vi "TcA01-008_NameObjectsWithUserCounter.vi"(1 "Input buffer":T3="1", 3 "Invocation info":T2, 5 "error in (no error)":errorcluster, 6 "Add log to result?":bool) -> (16 "Test Data":T1 {"Numeric Measurement" format="%.2f"}, 19 "error out":errorcluster)   [LabVIEW 2009]
doc: "Test case template."
uses:
  Shared/Support_InputBuffer.ctl
  Shared/Support_InvocationInfo.ctl
  Shared/Support_TestData.ctl
  <vilib>/addons/_AddQ/G#Object/utils/G#Object_CreateMethod.ctl
  TestClasses/G#BaseClass1_class/G#BaseClass1.lvclass
  TestClasses/G#SubClass1_class/G#SubClass1.lvclass
  <vilib>/addons/_AddQ/G#Object/G#Object.lvclass
panel:
  in  "Test name":string="TcA01-008 Name Objects With User Counter"
  out "Test result":bool
  out "Result":string
  # "Verify that objects can be named by a user counter."
  # "Sub test case"
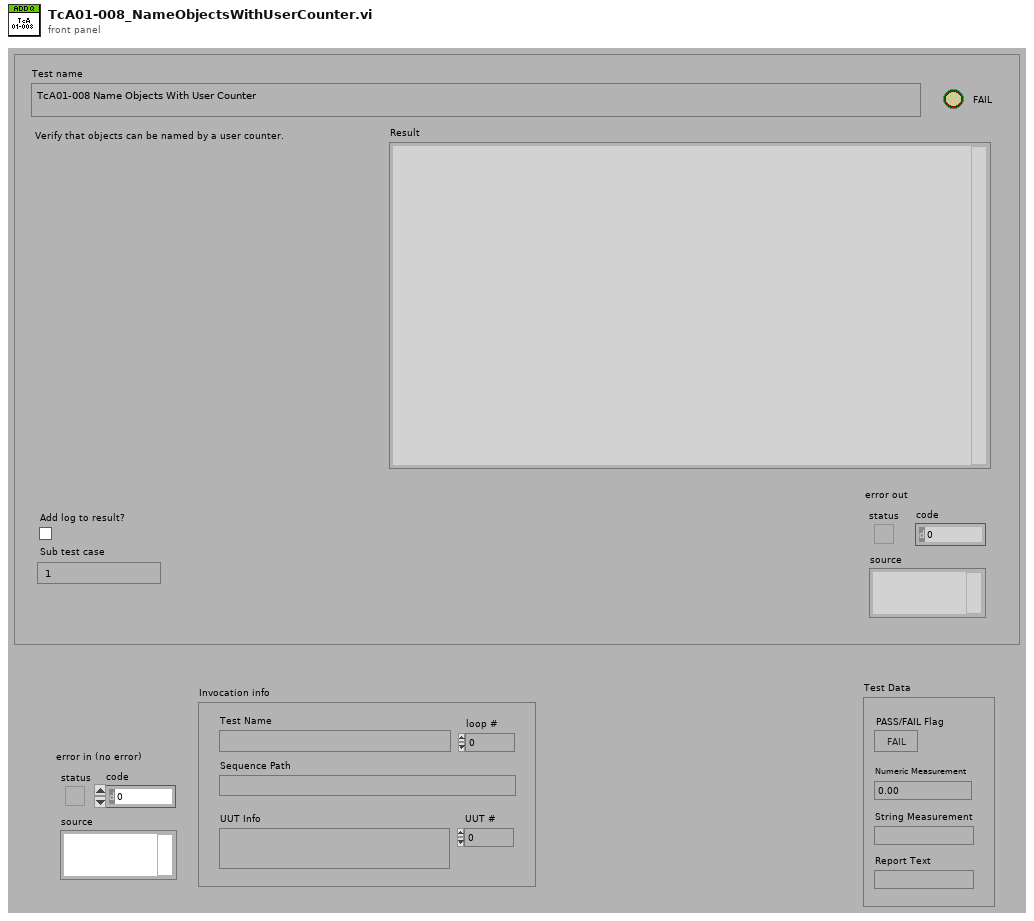
[diagram p1: front panel]
types:
  T1 = typedef "Support_TestData.ctl" = cluster{"PASS/FAIL Flag":bool, "Numeric Measurement":dbl, "String Measurement":string, "Report Text":string}
  T2 = typedef "Support_InvocationInfo.ctl" = cluster{"UUT #":i32, "loop #":i32, "UUT Info":string, "Test Name":string, "Sequence Path":path}
  T3 = typedef "Support_InputBuffer.ctl" = string
  T4 = typedef "G#Object.lvclass/G#Object_CreateMethod.ctl" = enum16{"Create", "Create or look up existing", "Look up existing"}
  T5 = typedef "Support_ResultType.ctl" = cluster{"Pass":bool, "Comment":string, "MeasurementValue":dbl}
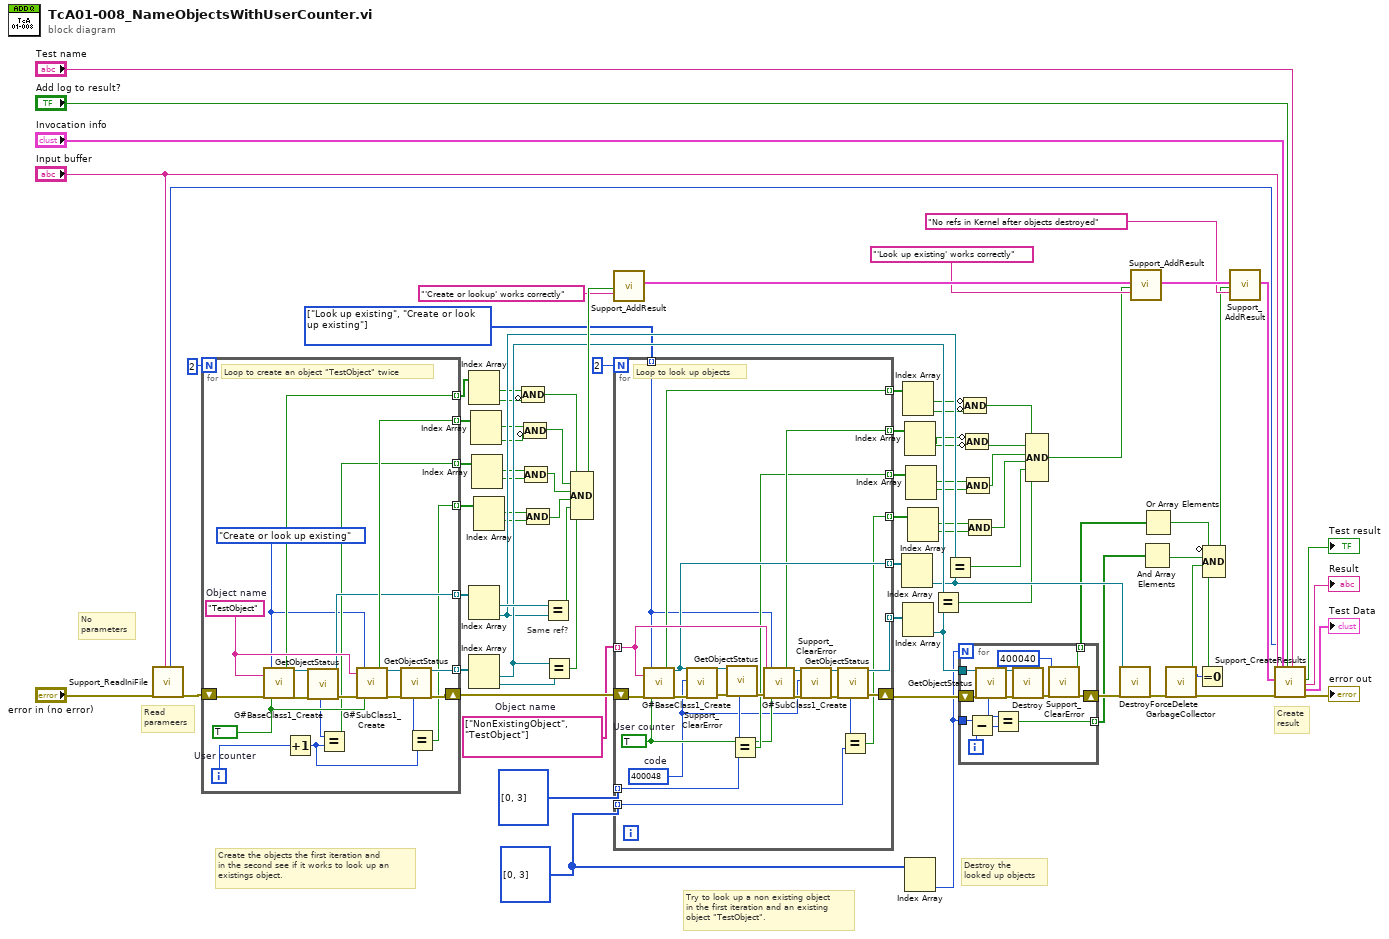
[diagram p0: block diagram]
diagram:
  w17 = T4[] [enum."Look up existing", enum."Create or look up existing"] items=["Create", "Create or look up existing", "Look up existing"]
  w11 = i32[] [0, 3]
  w31 = string[] ["NonExistingObject", "TestObject"]  # Object name
  # "Create the objects the first iteration and\nin the second see if it works to look up an\nexistings object."
  # "Try to look up a non existing object\nin the first iteration and an existing\nobject \"TestObject\"."
  # "Destroy the\nlooked up objects"
  # "Same ref?"
  # "No\nparameters"
  # "Create\nresult"
  # "Read\nparameers"
  n1 = call "Support_ReadIniFile.vi"("error in (no error)"="error in (no error)", "Sub test case"="Input buffer") -> ("Timer start"=w72:u32, "error out"=w71:errorcluster)  [unwired: 10 in, 6 out]
  n2 = for {
    N: 2 -> [_]
    shift-right: [w89] -> w57
    shift-left: w71 -> [w101]
    tunnel: [w94] -> w69 mode=indexing
    tunnel: [w90] -> w68 mode=indexing
    tunnel: [w98] -> w44 mode=indexing
    tunnel: [w97] -> w43 mode=indexing
    tunnel: [w86] -> w38 mode=indexing
    tunnel: [w83] -> w37 mode=indexing
    i -> [w87]
    w82 = G#Object_CreateMethod."Create or look up existing" ("create method")
    w99 = TRUE  # User counter
    w100 = "TestObject"  # Object name
    # "Loop to create an object \"TestObject\" twice"
    n3 = call "G#BaseClass1_Create.vi"("object name"=w100, "error in (no error)"=w101, "create method"=w82, "user counter"=w99) -> ("created new?"=w98:bool, "reference out"=w95:refnum<class "G#BaseClass1.lvclass">, "error out"=w96:errorcluster)  [unwired: 13 in]
    n4 = Increment(x=w87) -> (x+1=w84:i32)
    n5 = call-dynamic "GetObjectStatus.vi"("reference in"=w95, "error in (no error)"=w96) -> ("# of users?"=w88:i32, "reference out"=w94:refnum<class "G#BaseClass1.lvclass">, "error out"=w93:errorcluster)  [unwired: 6 in, 9 out]
    n6 = Equal?(x=w88, y=w84) -> (x = y?=w86:bool)
    n7 = call "G#SubClass1_Create.vi"("object name"=w100, "error in (no error)"=w93, "create method"=w82, "user counter"=w99) -> ("created new?"=w97:bool, "reference out"=w91:refnum<class "G#SubClass1.lvclass">, "error out"=w92:errorcluster)  [unwired: 13 in]
    n8 = call-dynamic "GetObjectStatus.vi"("reference in"=w91, "error in (no error)"=w92) -> ("# of users?"=w85:i32, "reference out"=w90:refnum<class "G#SubClass1.lvclass">, "error out"=w89:errorcluster)  [unwired: 6 in, 9 out]
    n9 = Equal?(x=w85, y=w84) -> (x = y?=w83:bool)
  }
  n10 = Index Array(array=w44) -> (element #1=w42:bool, element #2=w41:bool)  [unwired: 2 in]
  n11 = Index Array(array=w69) -> (element #1=w67:refnum<class "G#BaseClass1.lvclass">, element #2=w47:refnum<class "G#BaseClass1.lvclass">)  [unwired: 2 in]
  n12 = Index Array(array=w68) -> (element #1=w49:refnum<class "G#SubClass1.lvclass">, element #2=w66:refnum<class "G#SubClass1.lvclass">)  [unwired: 2 in]
  n13 = Index Array(array=w43) -> (element #1=w15:bool, element #2=w14:bool)  [unwired: 2 in]
  n14 = Index Array(array=w38) -> (element #1=w40:bool)  [unwired: 2 in, 1 out]
  n15 = Index Array(array=w37) -> (element #1=w39:bool)  [unwired: 2 in, 1 out]
  n16 = Compound Arithmetic op=AND(w42, invert w41) -> (w36:bool)
  n17 = Compound Arithmetic op=AND(w15, invert w14) -> (w35:bool)
  n18 = Compound Arithmetic op=AND(w40, w40) -> (w33:bool)
  n19 = Compound Arithmetic op=AND(w39, w39) -> (w32:bool)
  n20 = Equal?(x=w67, y=w47) -> (x = y?=w34:bool)
  n21 = Equal?(x=w49, y=w66) -> (x = y?=w65:bool)
  n22 = Compound Arithmetic op=AND(w36, w35, w33, w32, w34, w65) -> (w64:bool)
  n23 = call "Support_AddResult.vi"("Pass"=w64, "Comment"="'Create or lookup' works correctly") -> ("Results out"=w62:T5[])  [unwired: 17 in]
  n24 = for {
    N: 2 -> [_]
    shift-right: [w117] -> w53
    shift-left: w57 -> [w123]
    tunnel: [w119] -> w52 mode=indexing
    tunnel: [w115] -> w16 mode=indexing
    tunnel: w31 -> [w122] mode=indexing
    tunnel: [w113] -> w26 mode=indexing
    tunnel: [w112] -> w25 mode=indexing
    tunnel: [w111] -> w22 mode=indexing
    tunnel: [w110] -> w21 mode=indexing
    tunnel: i32[] [0, 3] -> [w109] mode=indexing
    tunnel: w11 -> [w108] mode=indexing
    tunnel: w17 -> [w106] mode=indexing
    w107 = TRUE  # User counter
    w103 = 400048  # code
    # "Loop to look up objects"
    n25 = call "G#BaseClass1_Create.vi"("object name"=w122, "error in (no error)"=w123, "create method"=w106, "user counter"=w107) -> ("created new?"=w113:bool, "reference out"=w119:refnum<class "G#BaseClass1.lvclass">, "error out"=w121:errorcluster)  [unwired: 13 in]
    n26 = call "Support_ClearError.vi"("code"=w103, "error in (no error)"=w121) -> ("error out"=w120:errorcluster)  [unwired: 16 in, 1 out]
    n27 = call-dynamic "GetObjectStatus.vi"("reference in"=w119, "error in (no error)"=w120) -> ("# of users?"=w116:i32, "error out"=w118:errorcluster)  [unwired: 6 in, 10 out]
    n28 = Equal?(x=w116, y=w109) -> (x = y?=w111:bool)
    n29 = call "G#SubClass1_Create.vi"("object name"=w122, "error in (no error)"=w118, "create method"=w106, "user counter"=w107) -> ("created new?"=w112:bool, "reference out"=w102:refnum<class "G#SubClass1.lvclass">, "error out"=w104:errorcluster)  [unwired: 13 in]
    n30 = call "Support_ClearError.vi"("code"=w103, "error in (no error)"=w104) -> ("error out"=w105:errorcluster)  [unwired: 16 in, 1 out]
    n31 = call-dynamic "GetObjectStatus.vi"("reference in"=w102, "error in (no error)"=w105) -> ("# of users?"=w114:i32, "reference out"=w115:refnum<class "G#SubClass1.lvclass">, "error out"=w117:errorcluster)  [unwired: 6 in, 9 out]
    n32 = Equal?(x=w114, y=w108) -> (x = y?=w110:bool)
  }
  n33 = Index Array(array=w52) -> (element #2=w48:refnum<class "G#BaseClass1.lvclass">)  [unwired: 2 in, 1 out]
  n34 = Index Array(array=w26) -> (element #1=w27:bool, element #2=w28:bool)  [unwired: 2 in]
  n35 = Index Array(array=w16) -> (element #2=w10:refnum<class "G#SubClass1.lvclass">)  [unwired: 2 in, 1 out]
  n36 = Index Array(array=w25) -> (element #1=w13:bool, element #2=w12:bool)  [unwired: 2 in]
  n37 = Index Array(array=w11) -> (element #2=w9:i32)  [unwired: 2 in, 1 out]
  n38 = Index Array(array=w22) -> (element #1=w29:bool)  [unwired: 2 in, 1 out]
  n39 = Index Array(array=w21) -> (element #1=w30:bool)  [unwired: 2 in, 1 out]
  n40 = Equal?(x=w49, y=w10) -> (x = y?=w45:bool)
  n41 = Equal?(x=w47, y=w48) -> (x = y?=w46:bool)
  n42 = for {
    N: w9 -> [_]
    shift-right: [w131] -> w54
    shift-left: w53 -> [w133]
    tunnel: w10 -> [w134]
    tunnel: w9 -> [w129]
    tunnel: [w125] -> w8 mode=indexing
    tunnel: [w124] -> w7 mode=indexing
    i -> [w130]
    n43 = Subtract(x=w129, y=w130) -> (x-y=w128:i32)
    n44 = call-dynamic "GetObjectStatus.vi"("reference in"=w134, "error in (no error)"=w133) -> ("# of users?"=w127:i32, "reference out"=w136:refnum<class "G#SubClass1.lvclass">, "error out"=w135:errorcluster)  [unwired: 6 in, 9 out]
    n45 = Equal?(x=w127, y=w128) -> (x = y?=w124:bool)
    n46 = call-dynamic "Destroy.vi"("reference in"=w136, "error in (no error)"=w135) -> ("error out"=w132:errorcluster)  [unwired: 16 in, 1 out]
    n47 = call "Support_ClearError.vi"("code"=400040, "error in (no error)"=w132) -> ("Cleared?"=w125:bool, "error out"=w131:errorcluster)  [unwired: 16 in]
  }
  n48 = Compound Arithmetic op=AND(invert w27, invert w28) -> (w24:bool)
  n49 = Compound Arithmetic op=AND(invert w13, invert w12) -> (w23:bool)
  n50 = Compound Arithmetic op=AND(w29, w29) -> (w20:bool)
  n51 = Compound Arithmetic op=AND(w30, w30) -> (w19:bool)
  n52 = Compound Arithmetic op=AND(w24, w23, w20, w19, w46, w45) -> (w51:bool)
  n53 = call-dynamic "DestroyForceDelete.vi"("reference in"=w48, "error in (no error)"=w54) -> ("error out"=w55:errorcluster)  [unwired: 16 in, 1 out]
  n54 = call "Support_AddResult.vi"("Results in"=w62, "Pass"=w51, "Comment"="'Look up existing' works correctly") -> ("Results out"=w61:T5[])  [unwired: 16 in]
  n55 = And Array Elements(Boolean array=w7) -> (logical AND=w6:bool)
  n56 = Or Array Elements(Boolean array=w8) -> (logical OR=w5:bool)
  n57 = call <vilib>:"GarbageCollector.vi"("error in (no error)"=w55) -> ("OK"=w4:bool, "# of objects killed"=w2:i32, "error out"=w58:errorcluster)  [unwired: 16 in]
  n58 = Equal To 0?(x=w2) -> (x = 0?=w1:bool)
  n59 = Compound Arithmetic op=AND(invert w5, w6, w4, w1) -> (w3:bool)
  n60 = call "Support_AddResult.vi"("Results in"=w61, "Pass"=w3, "Comment"="No refs in Kernel after objects destroyed") -> ("Results out"=w60:T5[])  [unwired: 16 in]
  n61 = call "Support_CreateResults.vi"("Sub test case"="Input buffer", "Timer start"=w72, "Results"=w60, "error in (no error)"=w58, "Invocation info"="Invocation info", "Add log to result?"="Add log to result?", "Test name"="Test name") -> ("Pass/fail flag"=→"Test result":bool, "Result"=→"Result":string, "Test Data"=→"Test Data":T1, "error out"=→"error out":errorcluster)  [unwired: 9 in]
